vi "Temperature Monitor.vi"() -> ()   [LabVIEW 2011]
panel:
  out "Elapsed Time (s)":dbl
  in  "Timer":bool caption="Reset"
  in  "Date format":enum16{"short", "long", "abbreviated"}(ring)
  in  "File Path":path
  out "size (in bytes)":i64
  out "Sorb":cluster{dbl[], dbl[]}(graph)
  out "3He pot":cluster{dbl[], dbl[]}(graph)
  out "current time":timestamp
  out "3HE Pot":string
  out "VTI":string
  out "Sorb":string
  out "Boolean":bool
  in  "Switch":bool
  in  "Time delay 2":dbl
  out "Warning":string="Can't be smaller than 1 s"
  in  "Heater":bool
  in  "Save":bool
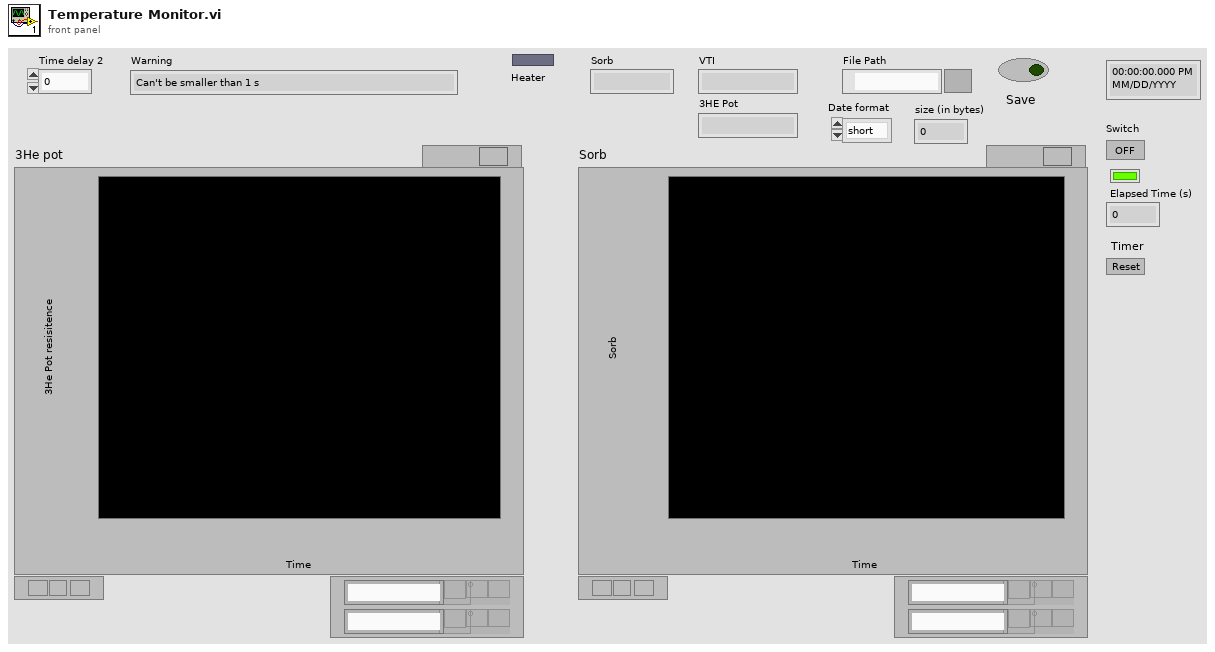
[diagram p1: front panel]
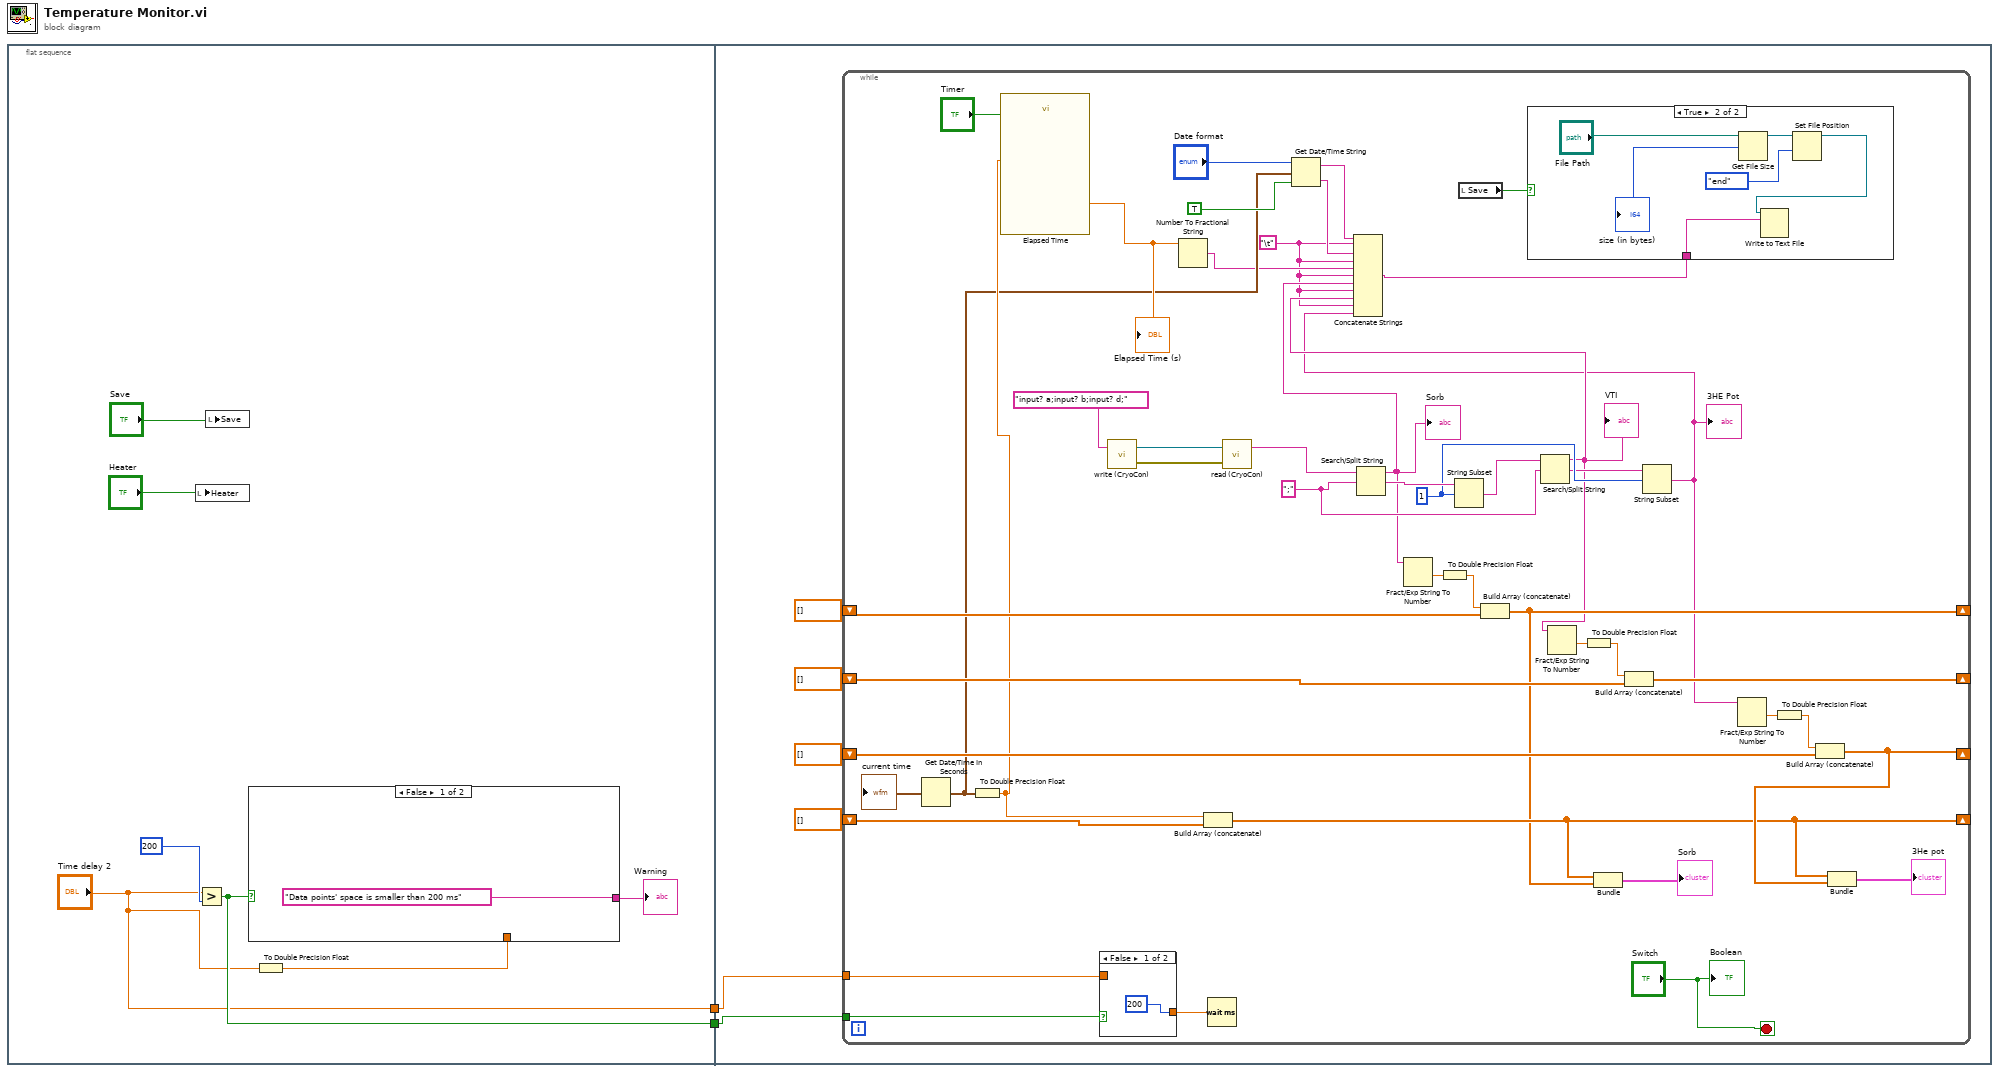
[diagram p0: block diagram]
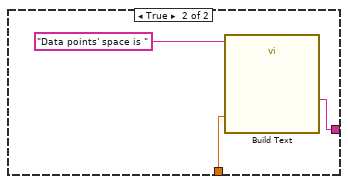
[diagram p2: hidden frame]
diagram:
  n1 = flat-sequence {
    tunnel: ["Time delay 2"] -> w2
    tunnel: [w4] -> w1
    tunnel: w2 -> [w18]
    tunnel: w1 -> [w19]
    frame #0 {
      n2 = local write "Heater"("Heater") -> ()
      n3 = Greater?(x="Time delay 2", y=u32 200 ("x")) -> (0:w4:bool)
      n4 = local write "Save"("Save") -> ()
      n5 = To Double Precision Float(number="Time delay 2") -> (double precision float=w5:dbl)
      n6 = case shown="False" w4 {
        tunnel: w5 -> [_ w11]
        tunnel: ["Data points' space is smaller than 200 ms" w13] -> w6
        frame False {
        }
        frame True {
          n7 = call "Build Text"("Beginning Text"="Data points' space is ", "Y"=w11) -> ("Result"=w13:string)  [unwired: 12 in, 1 out]
        }
      }
      "Warning" <- w6
    }
    frame #1 {
      n8 = while {
        tunnel: w19 -> [w62]
        tunnel: w18 -> [w61]
        shift-right: [w35] -> _
        shift-left: dbl[] [] -> [w48]
        shift-right: [w45] -> _
        shift-left: dbl[] [] -> [w44]
        shift-right: [w38] -> _
        shift-left: dbl[] [] -> [w40]
        shift-right: [w36] -> _
        shift-left: dbl[] [] -> [w41]
        stop <- "Switch" stop-if-true
        w21 = "\t"
        w52 = 1 ("offset (0)")
        w53 = ";" ("search string/char (-)")
        n9 = Get Date/Time In Seconds() -> (seconds since 1Jan1904=w27:timestamp)
        "current time" <- w27
        n10 = To Double Precision Float(number=w27) -> (double precision float=w28:dbl)
        n11 = call "Elapsed Time"("Reset"="Timer", "Set Start Time (s)"=w28) -> ("Elapsed Time (s)"=w30:dbl)  [unwired: 10 in, 7 out]
        "Elapsed Time (s)" <- w30
        n12 = case shown="False" w62 {
          tunnel: [200 w71] -> w63
          tunnel: w61 -> [_ w71]
          frame False {
          }
          frame True {
          }
        }
        n13 = call "write (CryoCon).vi"("write buffer"="input? a;input? b;input? d;") -> ("error out"=w59:errorcluster, "VISA resource name out"=w58:refnum<visa-resource-name>)  [unwired: 1 in]
        n14 = Number To Fractional String(number=w30) -> (F-format string=w24:string)  [unwired: 3 in]
        n15 = Build Array (concatenate)(w28, w41) -> (w36:dbl[])
        n16 = Wait (ms)(milliseconds to wait=w63) -> ()  [unwired: 1 out]
        n17 = call "read (CryoCon).vi"("error in (no error)"=w59, "VISA resource name"=w58) -> ("read buffer"=w55:string)  [unwired: 1 out]
        n18 = Get Date/Time String(date format (0)="Date format", seconds (now)=w27, want seconds? (F)=TRUE) -> (date string=w26:string, time string=w25:string)
        n19 = Search/Split String(string=w55, search string/char (-)=w53) -> (substring before match=w23:string, match + rest of string=w56:string)  [unwired: 1 in, 1 out]
        "Sorb" <- w23
        n20 = Fract/Exp String To Number(string=w23) -> (number=w50:dbl)  [unwired: 3 in, 1 out]
        n21 = To Double Precision Float(number=w50) -> (double precision float=w49:dbl)
        n22 = String Subset(string=w56, offset (0)=w52) -> (substring=w54:string)  [unwired: 1 in]
        n23 = local read "Save"() -> (w34:bool)
        n24 = Build Array (concatenate)(w49, w48) -> (w35:dbl[])
        n25 = Search/Split String(string=w54, search string/char (-)=w53) -> (substring before match=w22:string, match + rest of string=w51:string)  [unwired: 1 in, 1 out]
        "VTI" <- w22
        n26 = Fract/Exp String To Number(string=w22) -> (number=w47:dbl)  [unwired: 3 in, 1 out]
        n27 = To Double Precision Float(number=w47) -> (double precision float=w46:dbl)
        n28 = Bundle(w36, w35) -> (→"Sorb":cluster{dbl[], dbl[]})  [unwired: 1 in]
        n29 = Build Array (concatenate)(w46, w44) -> (w45:dbl[])
        n30 = String Subset(string=w51, offset (0)=w52) -> (substring=w20:string)  [unwired: 1 in]
        "3HE Pot" <- w20
        n31 = Concatenate Strings(w26, w21, w25, w21, w24, w21, w23, w21, w22, w21, w20) -> (w33:string)
        n32 = case shown="True" w34 {
          tunnel: w33 -> [_ w69]
          frame False {
          }
          frame True {
            n33 = Get File Size(file="File Path") -> (refnum out=w67:refnum<file>, size (in bytes)=→"size (in bytes)":i64)  [unwired: 1 in, 1 out]
            n34 = Set File Position(refnum=w67, from (0:start)=enum16{"start", "end", "current"}."end") -> (refnum out=w66:refnum<file>)  [unwired: 2 in, 1 out]
            n35 = Write to Text File(file (use dialog)=w66, text=w69) -> ()  [unwired: 2 in, 3 out]
          }
        }
        n36 = Fract/Exp String To Number(string=w20) -> (number=w43:dbl)  [unwired: 3 in, 1 out]
        n37 = To Double Precision Float(number=w43) -> (double precision float=w42:dbl)
        n38 = Build Array (concatenate)(w42, w40) -> (w38:dbl[])
        n39 = Bundle(w36, w38) -> (→"3He pot":cluster{dbl[], dbl[]})  [unwired: 1 in]
        "Boolean" <- "Switch"
      }
    }
  }
